vi "Service Stop Handler.vi"(8 "error in (no error)":errorcluster, 9 "Stop Server User Event":T1, 10 "Stop Button [ref]":refnum<vi>, 11 "IMeasurementService in":refnum<class "IMeasurement Service.lvclass">) -> (0 "error out":errorcluster, 3 "IMeasurementService out":refnum<class "IMeasurement Service.lvclass">)   [LabVIEW 2020, in "MeasurementLink Measurement Server.lvlib" / "IMeasurement Service.lvclass"]
uses:
  IMeasurement Service.lvclass
  Helpers/TypeDefs/Stop Server User Event.ctl
  MeasurementLink Measurement Server.lvlib
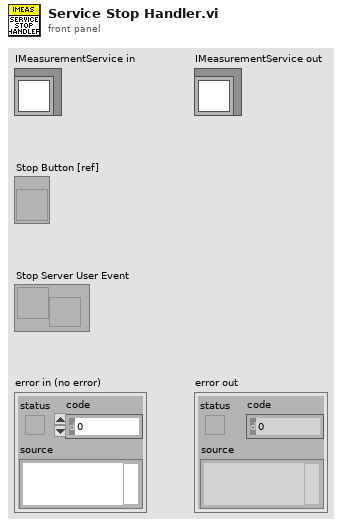
[diagram p1: front panel]
types:
  T1 = typedef "MeasurementLink Measurement Server.lvlib/Stop Server User Event.ctl" = refnum<user-event>
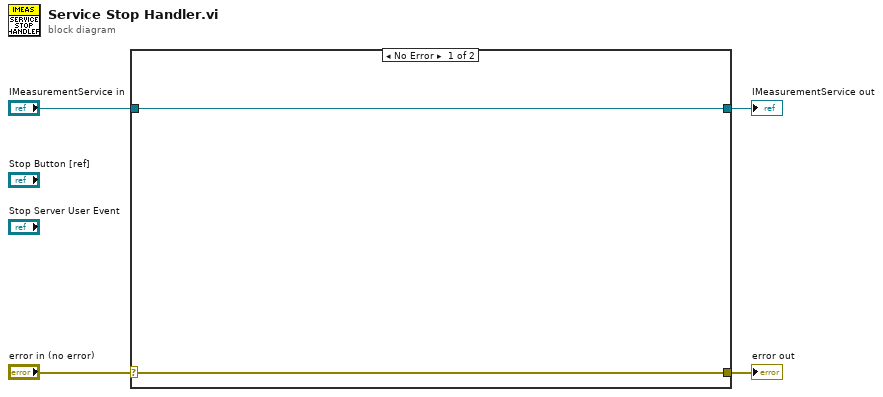
[diagram p0: block diagram]
diagram:
  n1 = case shown="No Error" "error in (no error)" {
    selector: "error in (no error)" -> [w5 w8]
    tunnel: [w5 w8] -> w3
    tunnel: [w6 w7] -> w1
    tunnel: "IMeasurementService in" -> [w6 w7]
    frame No Error {
    }
    frame Error {
    }
  }
  "error out" <- w3
  "IMeasurementService out" <- w1
